vi "Make DLL Param(Read Profile Req).vi"(1 "Read Profile Req":T3={"Read Area"=TRUE, "Profile Pos"=0, "Read Profile No."=0, "Read Profile Cnt"=0, "Erase"=FALSE} {"Profile Pos" items=["CURRENT", "OLDEST", "SPECIFY"]}) -> (0 "pReq":T2 {"Profile Pos" items=["CURRENT", "OLDEST", "SPECIFY"]})   [LabVIEW 2014, in "Keyence LJ-V7000.lvlib"]
uses:
  Keyence LJ-V7000.lvlib
  Public/Clusters/Read Profile Req.ctl
  Public/constant/Profile Pos.ctl
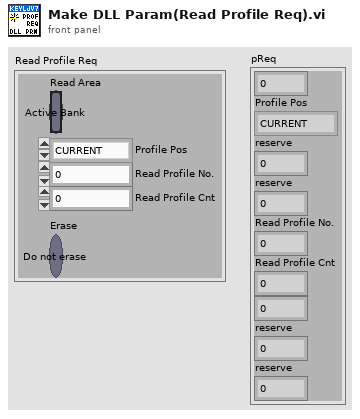
[diagram p1: front panel]
types:
  T1 = typedef "Keyence LJ-V7000.lvlib/Profile Pos.ctl" = u8
  T2 = cluster{u8, "Profile Pos":T1, "reserve":u8, "reserve":u8, "Read Profile No.":u32, "Read Profile Cnt":u8, u8, "reserve":u8, "reserve":u8}
  T3 = typedef "Keyence LJ-V7000.lvlib/Read Profile Req.ctl" = cluster{"Read Area":bool, "Profile Pos":T1, "Read Profile No.":u32, "Read Profile Cnt":u8, "Erase":bool}
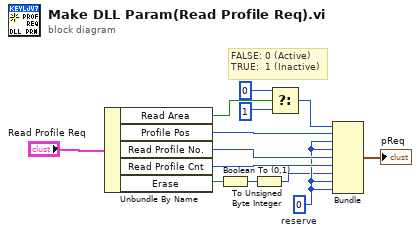
[diagram p0: block diagram]
diagram:
  w4 = u8 0  # reserve
  # "FALSE: 0 (Active)\nTRUE:  1 (Inactive)"
  n1 = Unbundle By Name("Read Profile Req") -> ("Read Area"=w12:bool, "Profile Pos"=w8:T1, "Read Profile No."=w7:u32, "Read Profile Cnt"=w6:u8, "Erase"=w5:bool)
  n2 = Boolean To (0,1)(Boolean=w5) -> (0, 1=w3:i16)
  n3 = To Unsigned Byte Integer(number=w3) -> (unsigned 8bit integer=w2:u8)
  n4 = Select(t=u8 0, s=w12, f=u8 1) -> (s? t:f=w9:u8)
  n5 = Bundle(w9, "Profile Pos"=w8, "reserve"=w4, "reserve"=w4, "Read Profile No."=w7, "Read Profile Cnt"=w6, w2, "reserve"=w4, "reserve"=w4) -> (→"pReq":T2)  [unwired: 1 in]
